vi "Set UI Busy State.vi"(7 "Defer Panel Updates":bool, 8 "error in (no error)":errorcluster, 11 "VI in":refnum<vi>) -> (0 "error out":errorcluster, 3 "VI out":refnum<vi>)   [LabVIEW 2017, in "DSF Mini Explorer.lvlib"]
uses:
  DSF Mini Explorer.lvlib
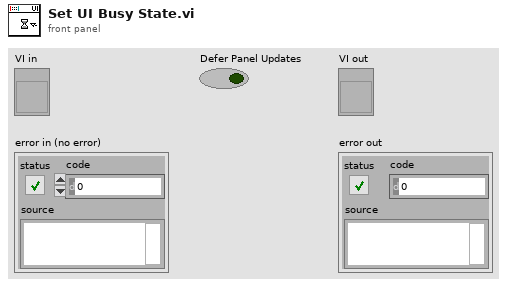
[diagram p1: front panel]
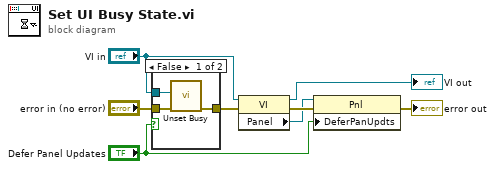
[diagram p0: block diagram]
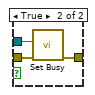
[diagram p2: hidden frame]
diagram:
  n1 = case shown="False" "Defer Panel Updates" {
    tunnel: "VI in" -> [w11 w14]
    tunnel: "error in (no error)" -> [w10 w13]
    tunnel: [w9 w12] -> w2
    frame False {
      n2 = call <vilib>:"Unset Busy.vi"("error in (no error)"=w10, "VI reference (current VI)"=w11) -> ("error out"=w9:errorcluster)  [unwired: 9 in]
    }
    frame True {
      n3 = call <vilib>:"Set Busy.vi"("error in (no error)"=w13, "VI reference (current VI)"=w14) -> ("error out"=w12:errorcluster)  [unwired: 8 in, 1 out]
    }
  }
  n4 = property class="VI"(reference="VI in", error in=w2) -> (reference out=→"VI out":refnum<vi>, error out=w7:errorcluster, "Panel"=w5:refnum<vi>)
  n5 = property class="Pnl"(reference=w5, error in=w7, "DeferPanUpdts"="Defer Panel Updates") -> (error out=→"error out":errorcluster)  [unwired: 1 out]
